vi "_PC_D999_STD.vi"(1 "index (row)":i32, 2 "Init? (F)":bool, 3 "new element/subarray":dbl[](array[numeric])) -> (0 "STD":dbl[](array[numeric]))   [LabVIEW 2018]
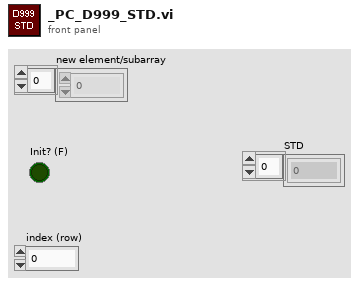
[diagram p1: front panel]
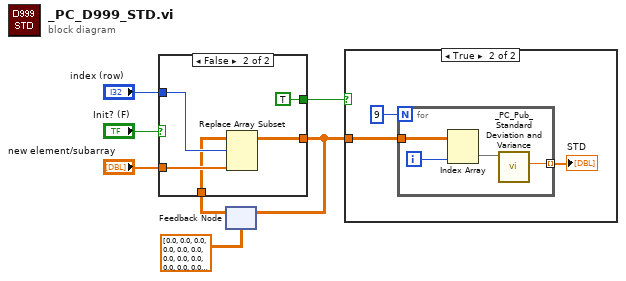
[diagram p0: block diagram]
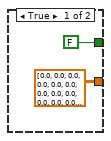
[diagram p3: hidden frame]
diagram:
  n1 = feedback #1(dbl[][] [[0.0, 0.0, 0.0, 0.0, 0.0, 0.0, 0.0, 0.0, 0.0], [0.0, 0.0, 0.0, 0.0, 0.0, 0.0, 0.0, 0.0, 0.0], [0.0, 0.0, 0.0, 0.0, 0.0, 0.0, 0.0, 0.0, 0.0], [0.0, 0.0, 0.0, 0.0, 0.0, 0.0, 0.0, 0.0, 0.0], [0.0, 0.0, 0.0, 0.0, 0.0, 0.0, 0.0, 0.0, 0.0], [0.0, 0.0, 0.0, 0.0, 0.0, 0.0, 0.0, 0.0, 0.0], [0.0, 0.0, 0.0, 0.0, 0.0, 0.0, 0.0, 0.0, 0.0], [0.0, 0.0, 0.0, 0.0, 0.0, 0.0, 0.0, 0.0, 0.0], [0.0, 0.0, 0.0, 0.0, 0.0, 0.0, 0.0, 0.0, 0.0]]) -> (w3:dbl[][])
  n2 = case shown="False" "Init? (F)" {
    tunnel: [dbl[][] [[0.0, 0.0, 0.0, 0.0, 0.0, 0.0, 0.0, 0.0, 0.0], [0.0, 0.0, 0.0, 0.0, 0.0, 0.0, 0.0, 0.0, 0.0], [0.0, 0.0, 0.0, 0.0, 0.0, 0.0, 0.0, 0.0, 0.0], [0.0, 0.0, 0.0, 0.0, 0.0, 0.0, 0.0, 0.0, 0.0], [0.0, 0.0, 0.0, 0.0, 0.0, 0.0, 0.0, 0.0, 0.0], [0.0, 0.0, 0.0, 0.0, 0.0, 0.0, 0.0, 0.0, 0.0], [0.0, 0.0, 0.0, 0.0, 0.0, 0.0, 0.0, 0.0, 0.0], [0.0, 0.0, 0.0, 0.0, 0.0, 0.0, 0.0, 0.0, 0.0], [0.0, 0.0, 0.0, 0.0, 0.0, 0.0, 0.0, 0.0, 0.0]] w14] -> w4
    tunnel: "new element/subarray" -> [_ w13]
    tunnel: "index (row)" -> [_ w12]
    tunnel: w3 -> [_ w11]
    tunnel: [FALSE TRUE] -> w2
    frame True {
    }
    frame False {
      n3 = Replace Array Subset(array=w11, new element=w13, index (row)=w12) -> (w14:dbl[][])  [unwired: 1 in]
    }
  }
  n4 = feedback-in #1(w4) -> ()
  n5 = case shown="True" w2 {
    tunnel: w4 -> [_ w15]
    frame False {
    }
    frame True {
      n6 = for {
        N: 9 -> [_]
        tunnel: w15 -> [w21]
        tunnel: [w18] -> w16 mode=indexing
        i -> [w20]
        n7 = Index Array(array=w21, index (col)=w20) -> (element=w19:dbl[])  [unwired: 1 in]
        n8 = call "_PC_Pub_Standard Deviation and Variance.vi"("X"=w19) -> ("standard deviation"=w18:dbl)  [unwired: 8 in, 2 out]
      }
      "STD" <- w16
    }
  }
